vi "JSON to LVObject - Unknown Type - Returns Error.vi"() -> ()   [LabVIEW 2017, in "Generic Object Serializer Tests.lvlib" / "Type Name Handling.lvlib"]
uses:
  Type Name Handling.lvlib
  Generic Object Serializer/Generic Object Serializer.lvclass
  Generic Object Serializer/Type Name Handling.ctl
  Generic Object Serializer/Generic Object Serializer.lvclass/Generic Object Serializer.ctl
  Generic Object Serializer/Write Type Name Handling.vi
  <vilib>/addons/_JKI Toolkits/Caraya/classes/Assert/Assert Error.vi
  <vilib>/addons/_JKI Toolkits/Caraya/classes/Test/Test.lvclass
  <vilib>/addons/_JKI Toolkits/Caraya/classes/Assert/Assert.lvclass
panel:
  out "error out":errorcluster
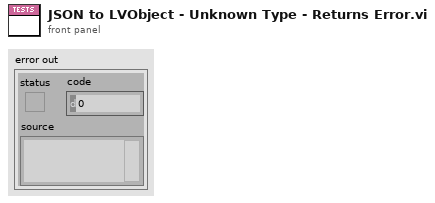
[diagram p1: front panel]
types:
  T1 = typedef "Generic Object Serializer.lvclass/Type Name Handling.ctl" = enum16{"None", "Inline"}
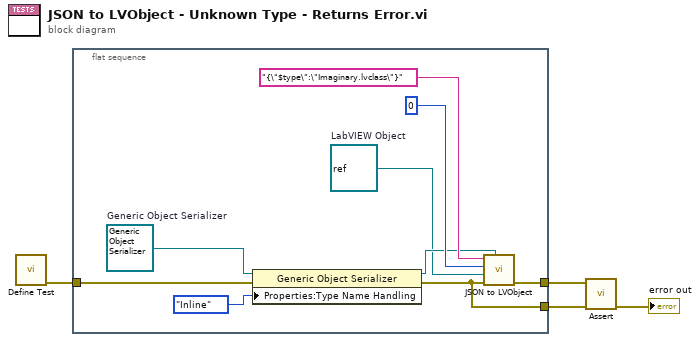
[diagram p0: block diagram]
diagram:
  n1 = call <vilib>:"Define Test.vi"() -> ("error out"=w4:errorcluster)  [unwired: 11 in]
  n2 = flat-sequence {
    tunnel: w4 -> [w13]
    tunnel: [w6] -> w2
    tunnel: [w5] -> w1
    frame #0 {
      w7 = refnum<class> refnum  # LabVIEW Object
      w10 = refnum<class "Generic Object Serializer.lvclass"> refnum  # Generic Object Serializer
      n3 = property class="Generic Object Serializer"(reference=w10, error in=w13, "Properties:Type Name Handling"=Type_Name_Handling."Inline" ("Type Name Handling")) -> (reference out=w9:refnum<class "Generic Object Serializer.lvclass">, error out=w5:errorcluster)
      n4 = call-dynamic "JSON to LVObject.vi"("LVClass Serializer"=w9, "error in (no error)"=w5, "Object Type"=w7, "Offset"=0, "JSON"="{\"$type\":\"Imaginary.lvclass\"}") -> ("error out"=w6:errorcluster)  [unwired: 5 in, 1 out]
    }
  }
  n5 = call-poly <vilib>:"Assert.vi"("error in (no error)"=w1, "Error?"=w2) -> ("error out"=→"error out":errorcluster)  [unwired: 9 in]
